vi "Queue In.vi"(7 "First":bool, 8 "error in (no error)":errorcluster caption="Error In", 9 "Data":variant, 10 "Message":string, 11 "Queue In":refnum<queue>) -> (0 "error out":errorcluster caption="Error Out", 3 "Queue Out":refnum<queue>)   [LabVIEW 2020]
uses:
  Queue Message.ctl
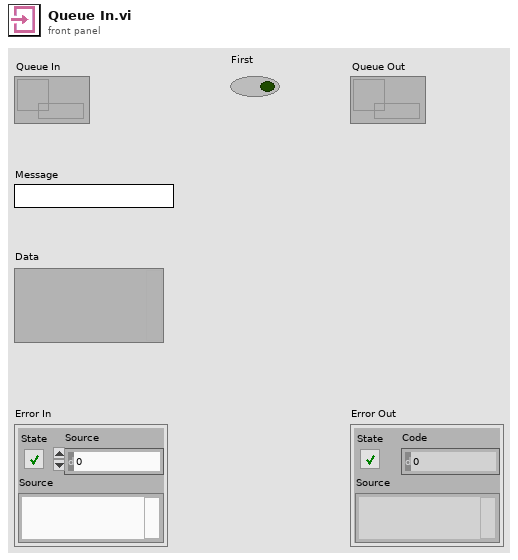
[diagram p1: front panel]
types:
  T1 = typedef "Queue Message.ctl" = cluster{"Message":string, "Data":variant}
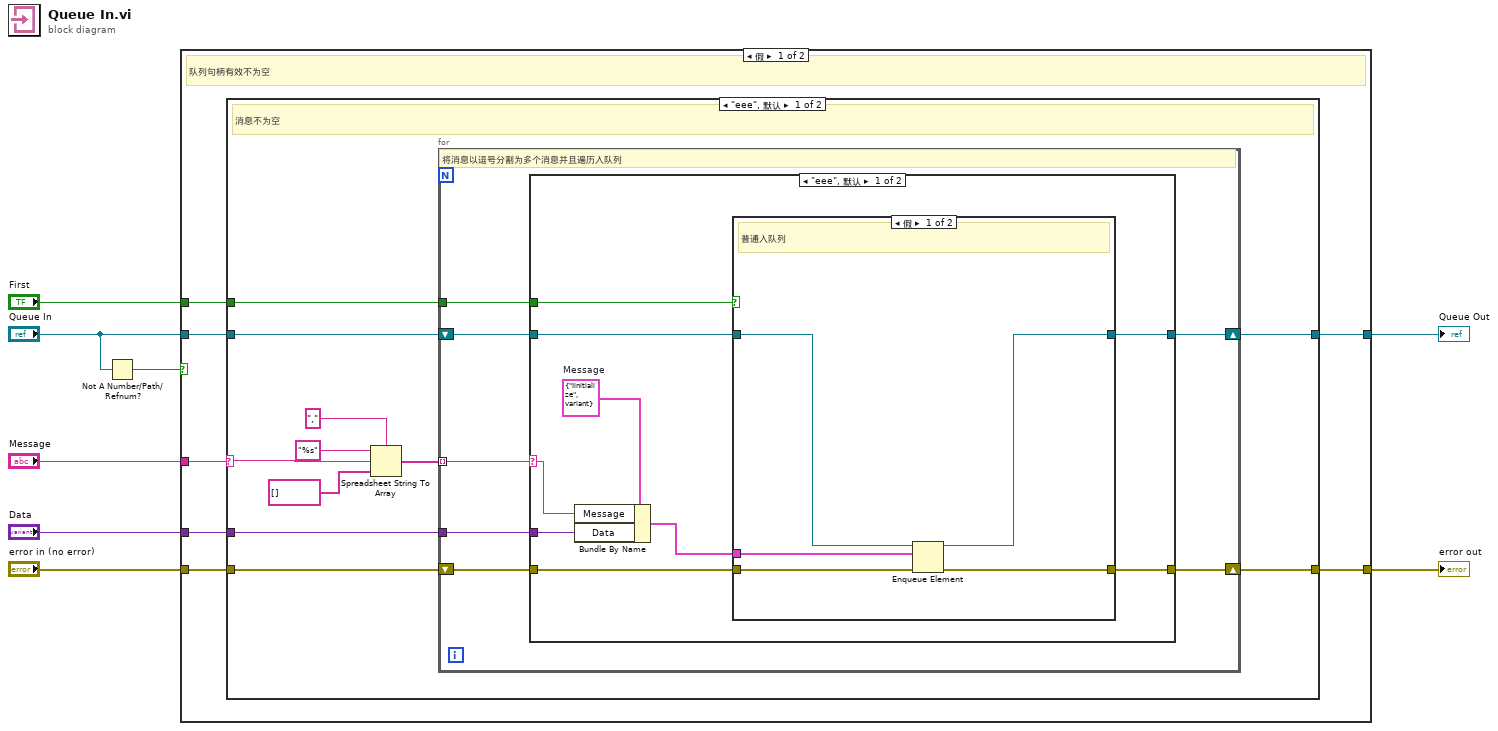
[diagram p0: block diagram]
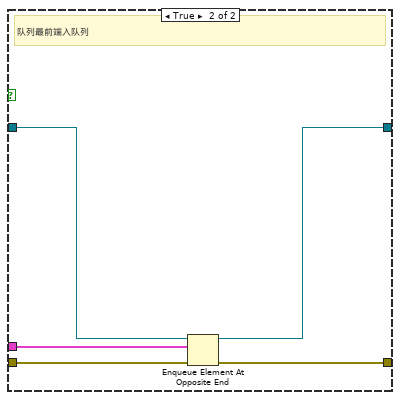
[diagram p2: hidden frame]
diagram:
  n1 = Not A Number/Path/Refnum?(number/path/refnum="Queue In") -> (NaN/Path/Refnum?=w1:bool)
  n2 = case shown="假" w1 {
    tunnel: [w15 w58] -> w8
    tunnel: "Data" -> [w14 _]
    tunnel: "error in (no error)" -> [w13 w57]
    tunnel: [w12 w57] -> w5
    tunnel: "First" -> [w11 _]
    tunnel: "Message" -> [w10 _]
    tunnel: "Queue In" -> [w9 w58]
    frame False {
      # "队列句柄有效不为空"
      n3 = case shown="\"eee\", 默认" w10 {
        selector: w10 -> [w18 _]
        tunnel: w9 -> [w26 w55]
        tunnel: [w25 w55] -> w15
        tunnel: w14 -> [w24 _]
        tunnel: w13 -> [w23 w56]
        tunnel: [w22 w56] -> w12
        tunnel: w11 -> [w21 _]
        frame "eee", Default {
          # "消息不为空"
          n4 = Spreadsheet String To Array(delimiter (Tab)="," ("分隔符(Tab)"), format string="%s" ("格式字符串"), spreadsheet string=w18, array type (2D Dbl)=string[] [] ("格式字符串")) -> (array=w17:string[])
          n5 = for {
            tunnel: w24 -> [w31]
            tunnel: w21 -> [w28]
            shift-right: [w32] -> w25
            shift-left: w26 -> [w33]
            shift-right: [w29] -> w22
            shift-left: w23 -> [w30]
            tunnel: w17 -> [w27] mode=indexing
            # "将消息以逗号分割为多个消息并且遍历入队列"
            n6 = case shown="\"eee\", 默认" w27 {
              selector: w27 -> [w34 _]
              tunnel: w33 -> [w36 w54]
              tunnel: [w38 w54] -> w32
              tunnel: w31 -> [w41 _]
              tunnel: w30 -> [w35 w53]
              tunnel: [w37 w53] -> w29
              tunnel: w28 -> [w40 _]
              frame "eee", Default {
                w39 = T1 {"Message"="Iinitialize", "Data"=variant}  # Message
                n7 = Bundle By Name(cluster=w39, "Message"=w34, "Data"=w41) -> (w42:T1)
                n8 = case shown="假" w40 {
                  tunnel: w36 -> [w47 w52]
                  tunnel: [w46 w49] -> w38
                  tunnel: w42 -> [w45 w48]
                  tunnel: w35 -> [w44 w51]
                  tunnel: [w43 w50] -> w37
                  frame False {
                    # "普通入队列"
                    n9 = Enqueue Element(queue=w47, element=w45, error in (no error)=w44) -> (queue out=w46:refnum<queue>, error out=w43:errorcluster)  [unwired: 1 in, 1 out]
                  }
                  frame True {
                    # "队列最前端入队列"
                    n10 = Enqueue Element At Opposite End(queue=w52, element=w48, error in (no error)=w51) -> (queue out=w49:refnum<queue>, error out=w50:errorcluster)  [unwired: 1 in, 1 out]
                  }
                }
              }
              frame "" {
              }
            }
          }
        }
        frame "" {
        }
      }
    }
    frame True {
    }
  }
  "Queue Out" <- w8
  "error out" <- w5
